vi "Unsupported Format Error.vi"(11 "Text Timestamp":string) -> (0 "Unsupported Format Error":errorcluster)   [LabVIEW 2024, in "JDP Timestamp.lvlib"]
uses:
  JDP Timestamp.lvlib
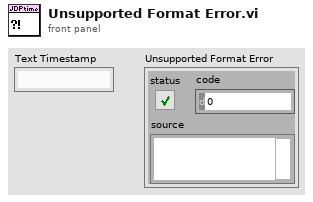
[diagram p1: front panel]
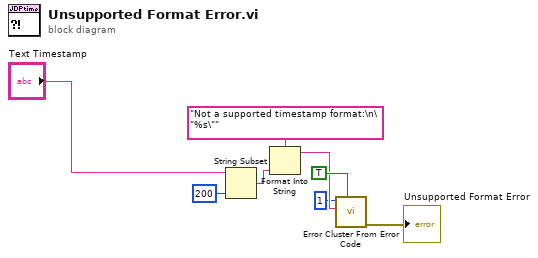
[diagram p0: block diagram]
diagram:
  n1 = String Subset(string="Text Timestamp", length (rest)=200 ("length (rest)")) -> (substring=w4:string)  [unwired: 1 in]
  n2 = Format Into String(format string="Not a supported timestamp format:\n\"%s\"", w4) -> (resulting string=w6:string)  [unwired: 2 in, 1 out]
  n3 = call "Error Cluster From Error Code.vi"("show call chain? (False)"=TRUE, "error message (\"\")"=w6, "error code (0)"=1) -> ("error out"=→"Unsupported Format Error":errorcluster)  [unwired: 6 in]
